vi "Advance Settings UI.vi"(0 "Advance Setting":T1, 11 "error in (no error)":errorcluster) -> (4 "Advance Setting Out":T1, 15 "error out":errorcluster)   [LabVIEW 2020, in "LDO Line Regulation.lvlib"]
uses:
  LDO Line Regulation.lvlib
  Reusables/Instrument APIs/Load Output Function.ctl
  Typedefs/Advance Settings.ctl
  <vilib>/Utility/error.llb/DialogType.ctl
  <userlib>/_Soliton/Measurement Suite/Reusables/Queue Driver/Plugin Queue Driver.lvlib
  <userlib>/_Soliton/Measurement Suite/Reusables/Plugin Common/Plugin Common.lvlib
panel:
  in  "CLOSE":bool
  in  "Initial Setup":cluster{"Output Function":T2}
  in  "Loop Delay (ms)":u32 caption="Delay between Stimulus and Measure (ms)" format="%#_6p"
  in  "Panel Close":bool
  out "Banner":picture caption="Advance Settings"
  # "For Each Voltage Sweep"
  # "Load SMU"
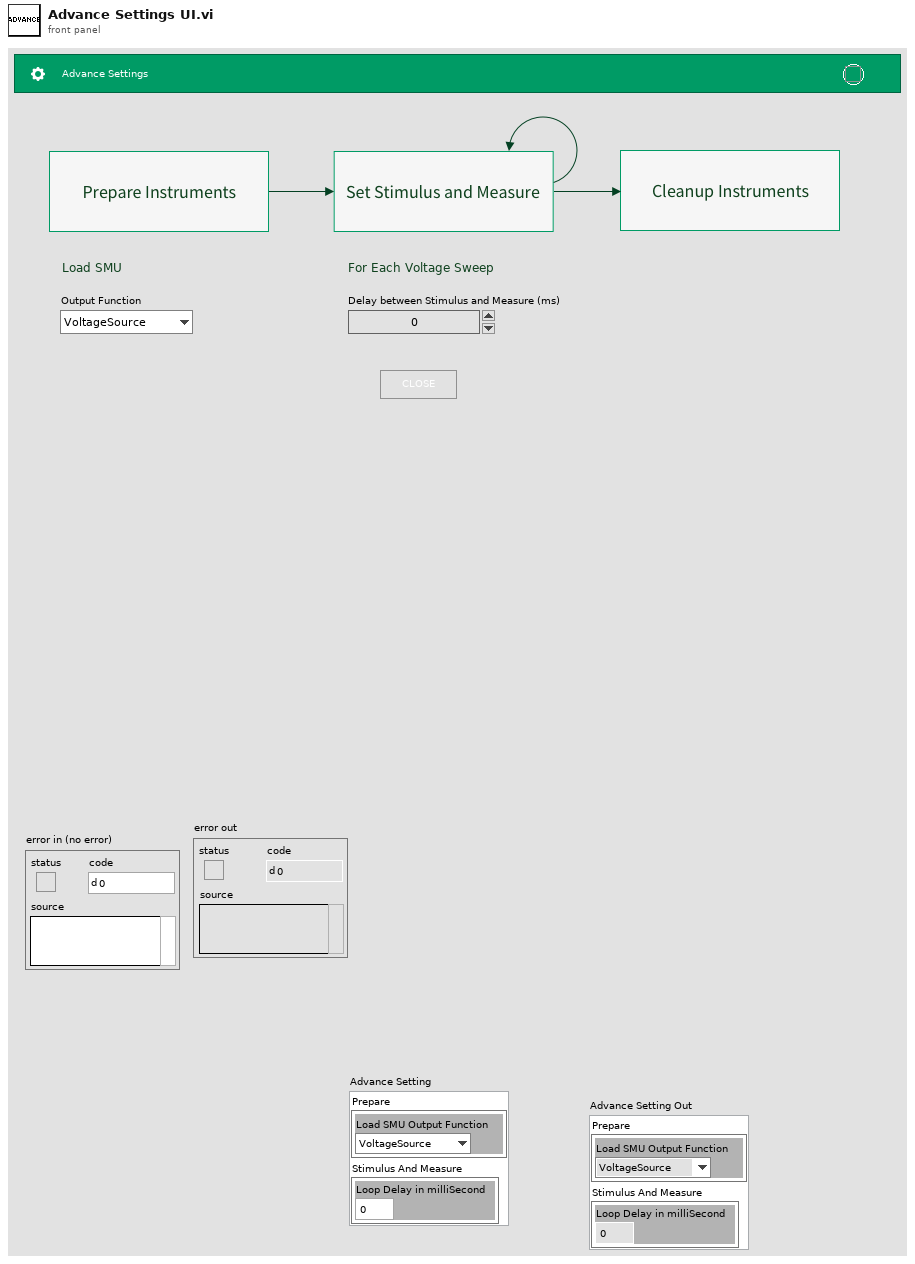
[diagram p1: front panel]
types:
  T1 = typedef "LDO Line Regulation.lvlib/Advance Settings.ctl" = cluster{"Prepare":cluster{"Load SMU Output Function":T2}, "Stimulus And Measure":cluster{"Loop Delay in milliSecond":u32}}
  T2 = typedef "Load Output Function.ctl" = enum16{"VoltageSource", "CurrentSource"}
  T3 = typedef "DialogType.ctl" = u16
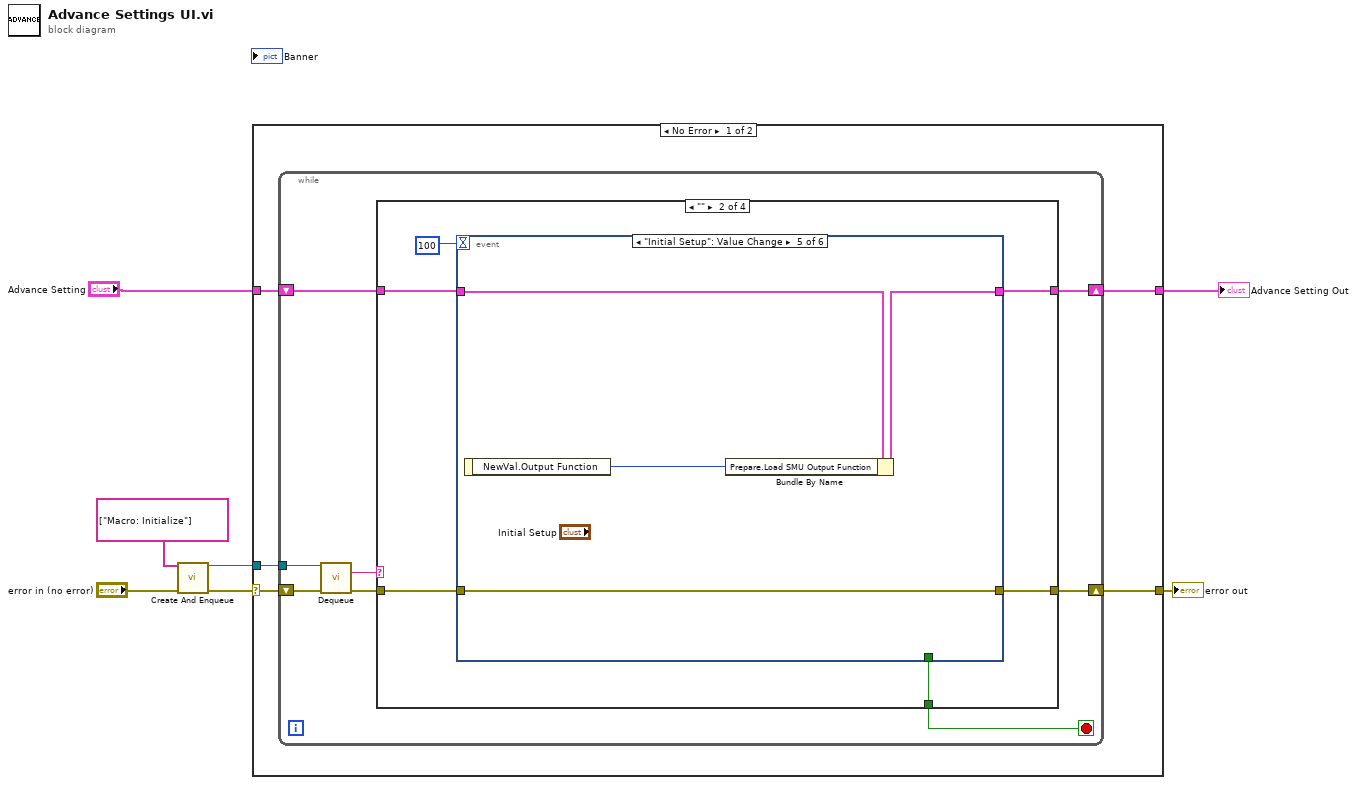
[diagram p0: block diagram]
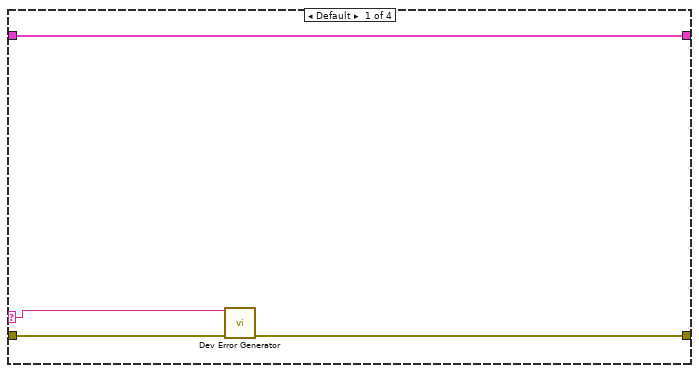
[diagram p2: hidden frame]
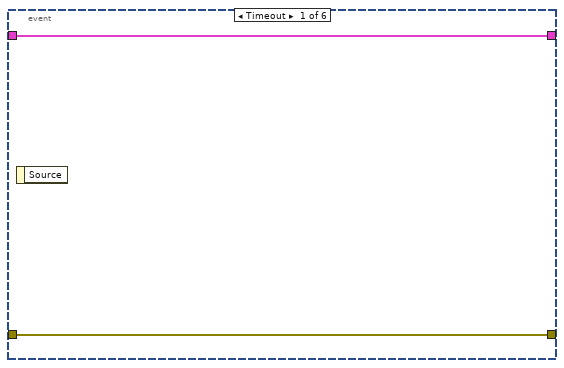
[diagram p3: hidden frame]
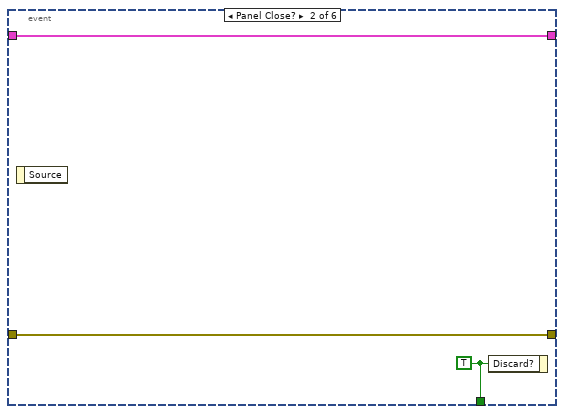
[diagram p4: hidden frame]
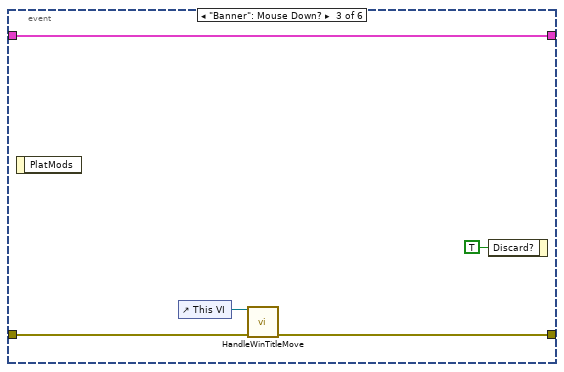
[diagram p5: hidden frame]
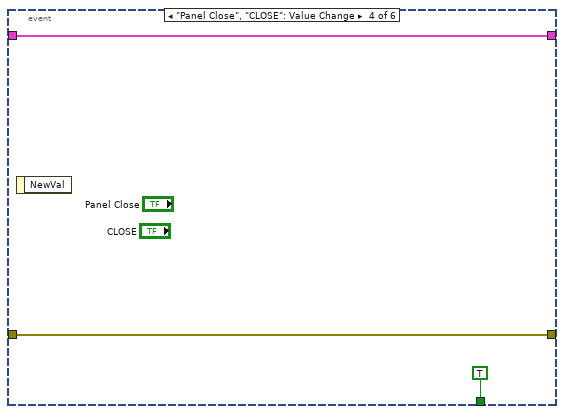
[diagram p6: hidden frame]
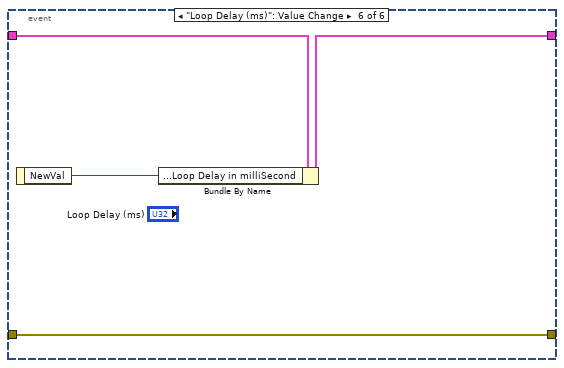
[diagram p7: hidden frame]
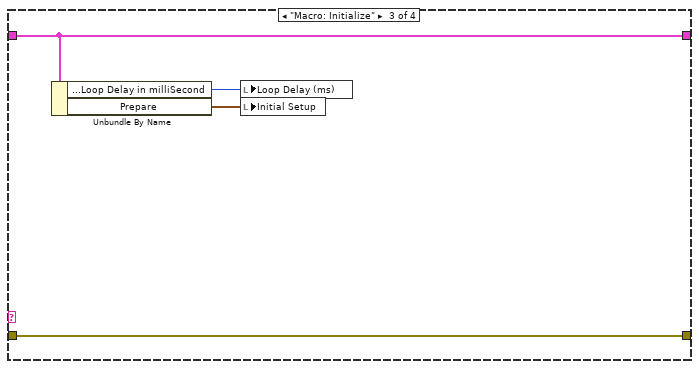
[diagram p8: hidden frame]
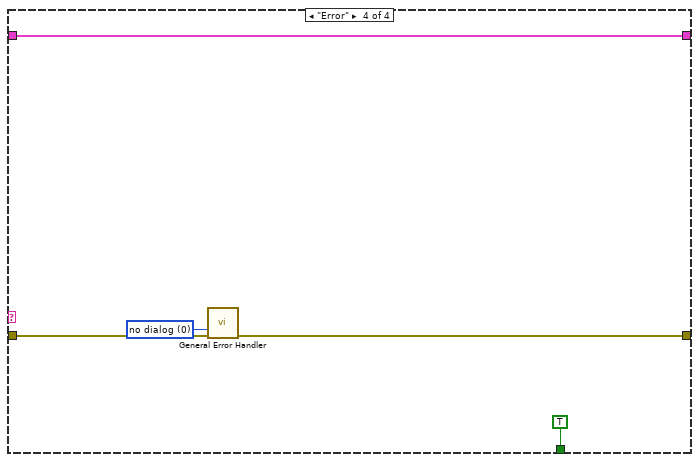
[diagram p9: hidden frame]
diagram:
  n1 = call <userlib>:"Create And Enqueue.vi"("Initial States"=string[] ["Macro: Initialize"], "error in (no error)"="error in (no error)") -> ("Queue out"=w4:refnum<queue>, "error out"=w5:errorcluster)  [unwired: 12 in]
  n2 = case shown="No Error" w5 {
    selector: w5 -> [w8 w62]
    tunnel: [w12 w62] -> w7
    tunnel: "Advance Setting" -> [w11 w61]
    tunnel: [w10 w61] -> w1
    tunnel: w4 -> [w9 _]
    frame No Error {
      n3 = while {
        tunnel: w9 -> [w17]
        shift-right: [w18] -> w10
        shift-left: w11 -> [w19]
        shift-right: [w20] -> w12
        shift-left: w8 -> [w16]
        stop <- w13 stop-if-true
        n4 = call <userlib>:"Dequeue.vi"("Queue in"=w17, "error in (no error)"=w16) -> ("Dequeued State"=w14:string, "error out"=w15:errorcluster)  [unwired: 11 in, 1 out]
        n5 = case shown="\"\"" w14 {
          selector: w14 -> [w21 _ _ _]
          tunnel: [w23 w30 w55 w58] -> w20
          tunnel: w19 -> [w24 w29 w54 w60]
          tunnel: [w24 w28 w54 w60] -> w18
          tunnel: w15 -> [w22 w27 w55 w57]
          tunnel: [_ w25 _ TRUE] -> w13
          frame Default {
            n6 = call <userlib>:"Dev Error Generator.vi"("State"=w21, "error in (no error)"=w22) -> ("error out"=w23:errorcluster)  [unwired: 13 in]
          }
          frame "" {
            n7 = event shown="[4] \"Initial Setup\": Value Change" {
              selector: _ -> [_ _ _ _ _ _]
              dyn-events: _ -> [_ _ _ _ _ _]
              timeout: 100 -> [_ _ _ _ _ _]
              tunnel: w27 -> [w32 w35 w37 w43 w47 w51]
              tunnel: [w32 w35 w38 w43 w47 w51] -> w30
              tunnel: [_ w33 _ TRUE _ _] -> w25
              tunnel: w29 -> [w31 w34 w40 w41 w45 w48]
              tunnel: [w31 w34 w40 w41 w46 w49] -> w28
              event Timeout {
                n8 = event-data() -> ()  [unwired: 1 in, 1 out]
              }
              event Panel Close? {
                w33 = TRUE ("Discard?")
                n9 = event-data() -> ()  [unwired: 1 in, 1 out]
                n10 = event-data("Discard?"=w33) -> ()  [unwired: 1 in, 1 out]
              }
              event "Banner": Mouse Down? {
                n11 = event-data() -> ()  [unwired: 1 in, 1 out]
                n12 = control-ref of="This VI"() -> (w36:refnum<vi>)
                n13 = call "HandleWinTitleMove.vi"("VI in"=w36, "error in (no error)"=w37) -> ("error out"=w38:errorcluster)  [unwired: 12 in, 1 out]
                n14 = event-data("Discard?"=TRUE) -> ()  [unwired: 1 in, 1 out]
              }
              event "Panel Close", "CLOSE": Value Change {
                n15 = event-data() -> ()  [unwired: 1 in, 1 out]
              }
              event "Initial Setup": Value Change {
                n16 = event-data() -> ("NewVal.Output Function"=w44:T2)  [unwired: 1 in]
                n17 = Bundle By Name(cluster=w45, "Prepare.Load SMU Output Function"=w44) -> (w46:T1)
              }
              event "Loop Delay (ms)": Value Change {
                n18 = event-data() -> ("NewVal"=w50:u32)  [unwired: 1 in]
                n19 = Bundle By Name(cluster=w48, "Stimulus And Measure.Loop Delay in milliSecond"=w50) -> (w49:T1)
              }
            }
          }
          frame "Macro: Initialize" {
            n20 = Unbundle By Name(w54) -> ("Stimulus And Measure.Loop Delay in milliSecond"=w53:u32, "Prepare"=w52:cluster{"Load SMU Output Function":T2})
            n21 = local write "Loop Delay (ms)"(w53) -> ()
            n22 = local write "Initial Setup"(w52) -> ()
          }
          frame "Error" {
            w59 = T3 0 items=["no dialog", "OK message", "continue or stop message", "OK message + warnings", "continue/stop + warnings"] ("type of dialog (OK msg:1)")
            n23 = call <vilib>:"General Error Handler.vi"("type of dialog (OK msg:1)"=w59, "error in (no error)"=w57) -> ("error out"=w58:errorcluster)  [unwired: 9 in, 4 out]
          }
        }
      }
    }
    frame Error {
    }
  }
  "error out" <- w7
  "Advance Setting Out" <- w1
